vi "Pre Launch Init.vi"(11 "ATM Controller in":refnum<class "ATM Controller.lvclass">) -> (0 "error out":errorcluster, 3 "ATM Controller out":refnum<class "ATM Controller.lvclass">)   [LabVIEW 2019, in "ATM Controller.lvlib" / "ATM Controller.lvclass"]
doc: "(<B>Filename</B>: Actor Framework.lvlib:Actor.lvclass:Pre Launch Init.vi)\n\nDefines behavior that occurs after the Launch Nested Actor method is invoked but before the actor's Actor Core method begins running.\n\nBy default, this method does nothing. A descendant class may override it to define behavior."
uses:
  ATM Controller.lvclass
  ATM Controller.lvclass/ATM Controller.ctl
  <vilib>/ActorFramework/Actor/Actor.lvclass
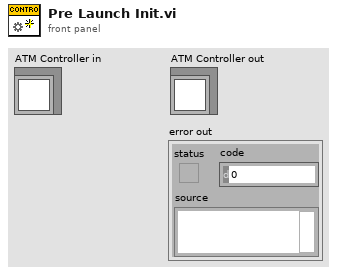
[diagram p1: front panel]
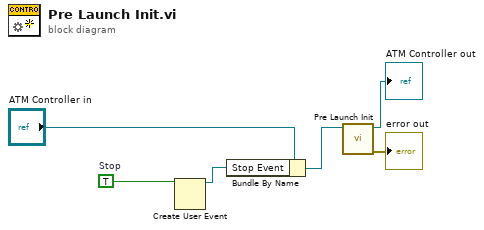
[diagram p0: block diagram]
diagram:
  w4 = TRUE  # Stop
  n1 = Create User Event(user event datatype=w4) -> (user event=w3:refnum<user-event>)  [unwired: 1 in, 1 out]
  n2 = Bundle By Name(cluster="ATM Controller in", "Stop Event"=w3) -> (w1:refnum<class "ATM Controller.lvclass">)
  n3 = call-parent "Pre Launch Init.vi"("Actor in"=w1) -> ("error out"=→"error out":errorcluster, "Actor out"=→"ATM Controller out":refnum<class "ATM Controller.lvclass">)  [unwired: 9 in]
